vi "梦幻城堡C6~20界面.vi"() -> ()   [LabVIEW 2016, in "环境动力监测库.lvlib" / "UPS库.lvlib"]
uses:
  <vilib>/Utility/config.llb/NI_LVConfig.lvlib
panel:
  out "x+1":u32
  in  "解除告警":bool
  out "状态":T1
  out "通信":bool=TRUE
  out "串口":string
  in  "查看型号":bool
  out "关闭中":bool
  out "关机倒计时":i32
  out "UPS状态":T2
  in  "关机":bool
  in  "重开串口":bool
  # "V"
  # "输入电压"
  # "输出电压"
  # "V"
  # "输出电流"
  # "A"
  # "Hz"
  # "输入频率"
  # "电池电压"
  # "V"
  # "℃"
  # "UPS温度"
  # "%"
  # "电池容量百分比"
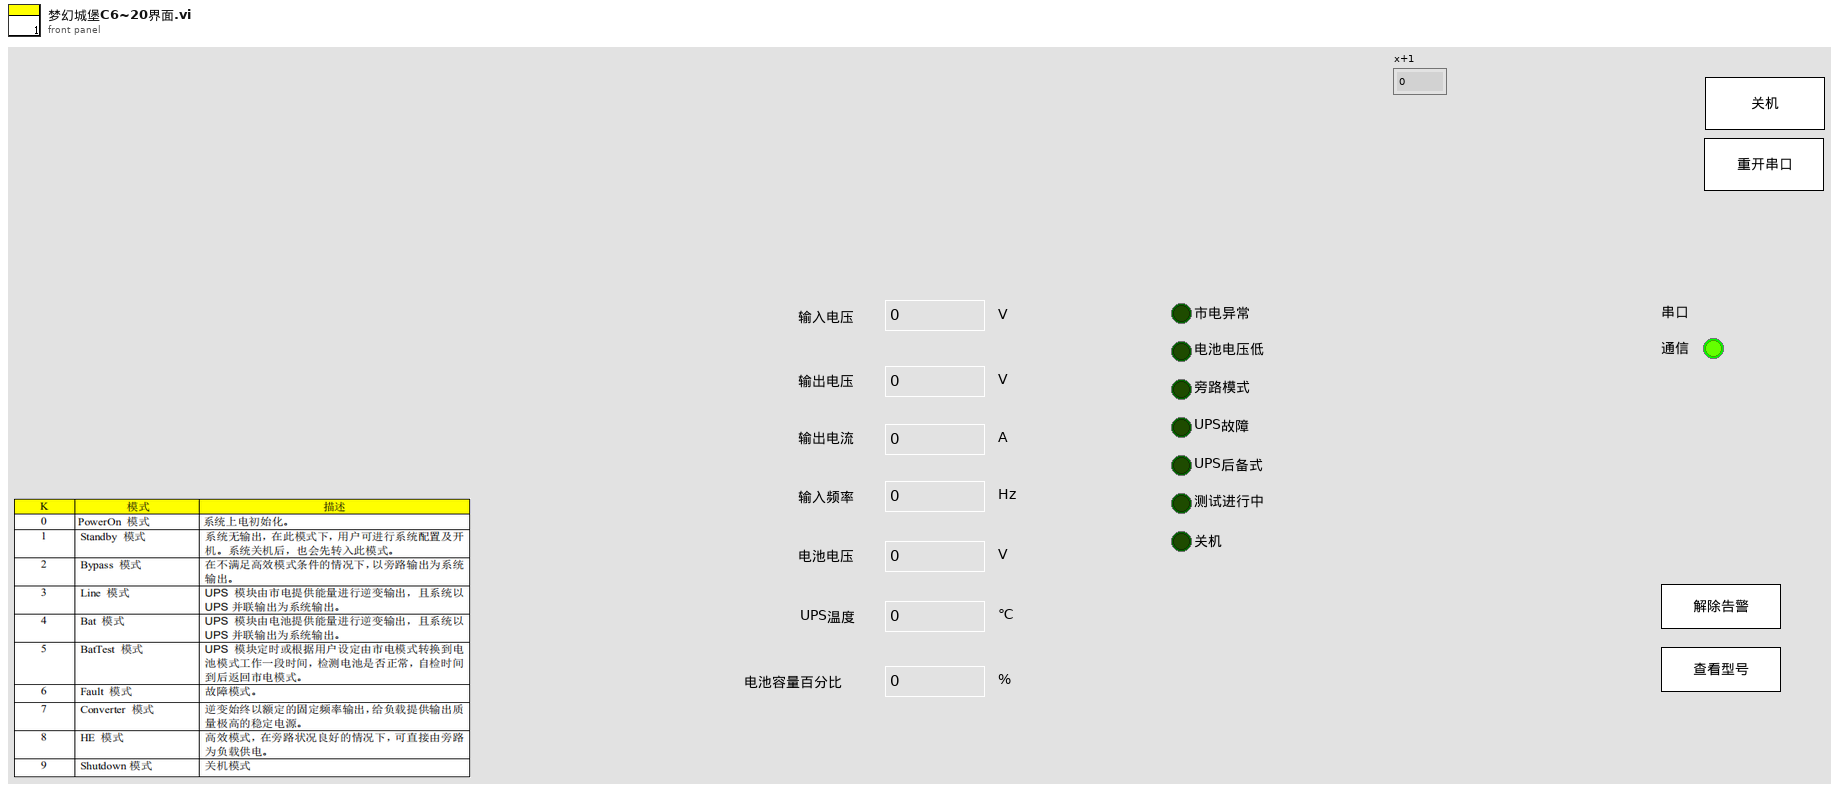
[diagram p1: front panel]
types:
  T1 = cluster{"I/P voltage":dbl, "O/P voltage":dbl, "O/P load %":dbl, "I/P frequency HZ":dbl, "Battery voltage":dbl, "Temperature":dbl, "CCC":dbl}
  T2 = cluster{"市电异常":bool, "电池电压低":bool, "旁路模式":bool, "UPS故障":bool, "UPS后备式":bool, "测试进行中":bool, "关机":bool, "保留":bool}
  T3 = cluster{"枚举":enum16{"open", "read", "write", "close"}, "写入缓冲区":string}
  T4 = cluster{"漏水监测输出":cluster{"漏水监测告警":bool, "告警内容":string}, "门禁监测输出":cluster{"门禁监测告警":bool, "告警内容":string}, "门禁监测输出2":cluster{"门禁监测告警":bool, "告警内容":string}, "温湿度监测输出":cluster{"温湿度监测告警":bool, "告警内容":string}, "烟雾监测输出":cluster{"烟雾监测告警":bool, "告警内容":string}, "空调监测输出":cluster{"空调监测告警":bool, "告警内容":string}, "自动重合闸输出":cluster{"自动重合闸告警":bool, "告警内容":string}, "红外入侵输出":cluster{"红外入侵告警":bool, "告警内容":string}, "振动输出":cluster{"振动告警":bool, "告警内容":string}, "UPS输出":cluster{"UPS告警":bool, "告警内容":string}, "蓄电池输出":cluster{"蓄电池告警":bool, "告警内容":string}, "蓄电池输出2":cluster{"蓄电池告警":bool, "告警内容":string}, "GPS输出":cluster{"定位告警":bool, "告警内容":string}, "北斗输出":cluster{"定位告警":bool, "告警内容":string}, "气象输出":cluster{"气象告警":bool, "告警内容":string}}
  T5 = cluster{"VISA resource name":refnum<visa-resource-name>, "Serial Config":cluster{"baud rate (9600)":u32, "stop bits (10: 1 bit)":u16, "parity (0:none)":enum16{"None", "Odd", "Even", "Mark", "Space"}, "data bits (8)":u16, "timeout (10sec)":u32}, "型号选择":enum16{"山特UPSC1~3", "山特UPSC6~20", "华为UPS2000-G-(1-3KVA)"}, "HW-UPS-2000 MB session":refnum<class "MB_Master.lvclass">, "连接方式":enum16{"串口", "TCP"}, "IP":string, "Port":string}
  T6 = typedef "NI_LVConfig.lvlib/Config Data RefNum.ctl" = refnum<k1>
  T7 = cluster{"输出功率R":dbl, "输出功率S":dbl, "输出功率T":dbl, "输出视在功率R":dbl, "输出视在功率S":dbl, "输出视在功率T":dbl, "总功率":dbl, "总视在功率":dbl, "输出电流R":dbl, "输出电流S":dbl, "输出电流T":dbl, "输出负载百分比":dbl, "U":string}
  T8 = cluster{"输入电压R":dbl, "输入电压S":dbl, "输入电压T":dbl, "输入频率":dbl, "输出电压R":dbl, "输出电压S":dbl, "输出电压T":dbl, "输出频率":dbl, "输出电流R":dbl, "输出电流S":dbl, "输出电流T":dbl, "Positive电池电压":dbl, "Negative电池电压":dbl, "温度":dbl, "电池剩余备用时间":dbl, "电池容量百分比":dbl, "系统模式":dbl, "电池测试状态":dbl, "故障代码":string, "告警":string}
  T9 = cluster{"市电":cluster{"状态":bool, "电压:":u16, "电流：":dbl, "详情  ":bool}, "UPS":cluster{"状态":bool, "输入电压:":sgl, "输出电压:":sgl, "电池电量:":u8, "电量":u16, "详情  ":bool}, "蓄电池12V":cluster{"状态":bool, "电压:":sgl, "电流:":sgl, "电池电量:":u8, "电量":u16, "详情  ":bool}, "蓄电池24V":cluster{"状态":bool, "电压:":sgl, "电流:":sgl, "电池电量:":u8, "电量":u16, "详情  ":bool}}
  T10 = cluster{"[0]":bool, "[1]":bool, "[2]":bool, "[3]":bool, "[4]":bool, "[5]":bool, "[6]":bool, "[7]":bool}
  T11 = enum32{"Bad", "Idle", "Run top level", "Running"}
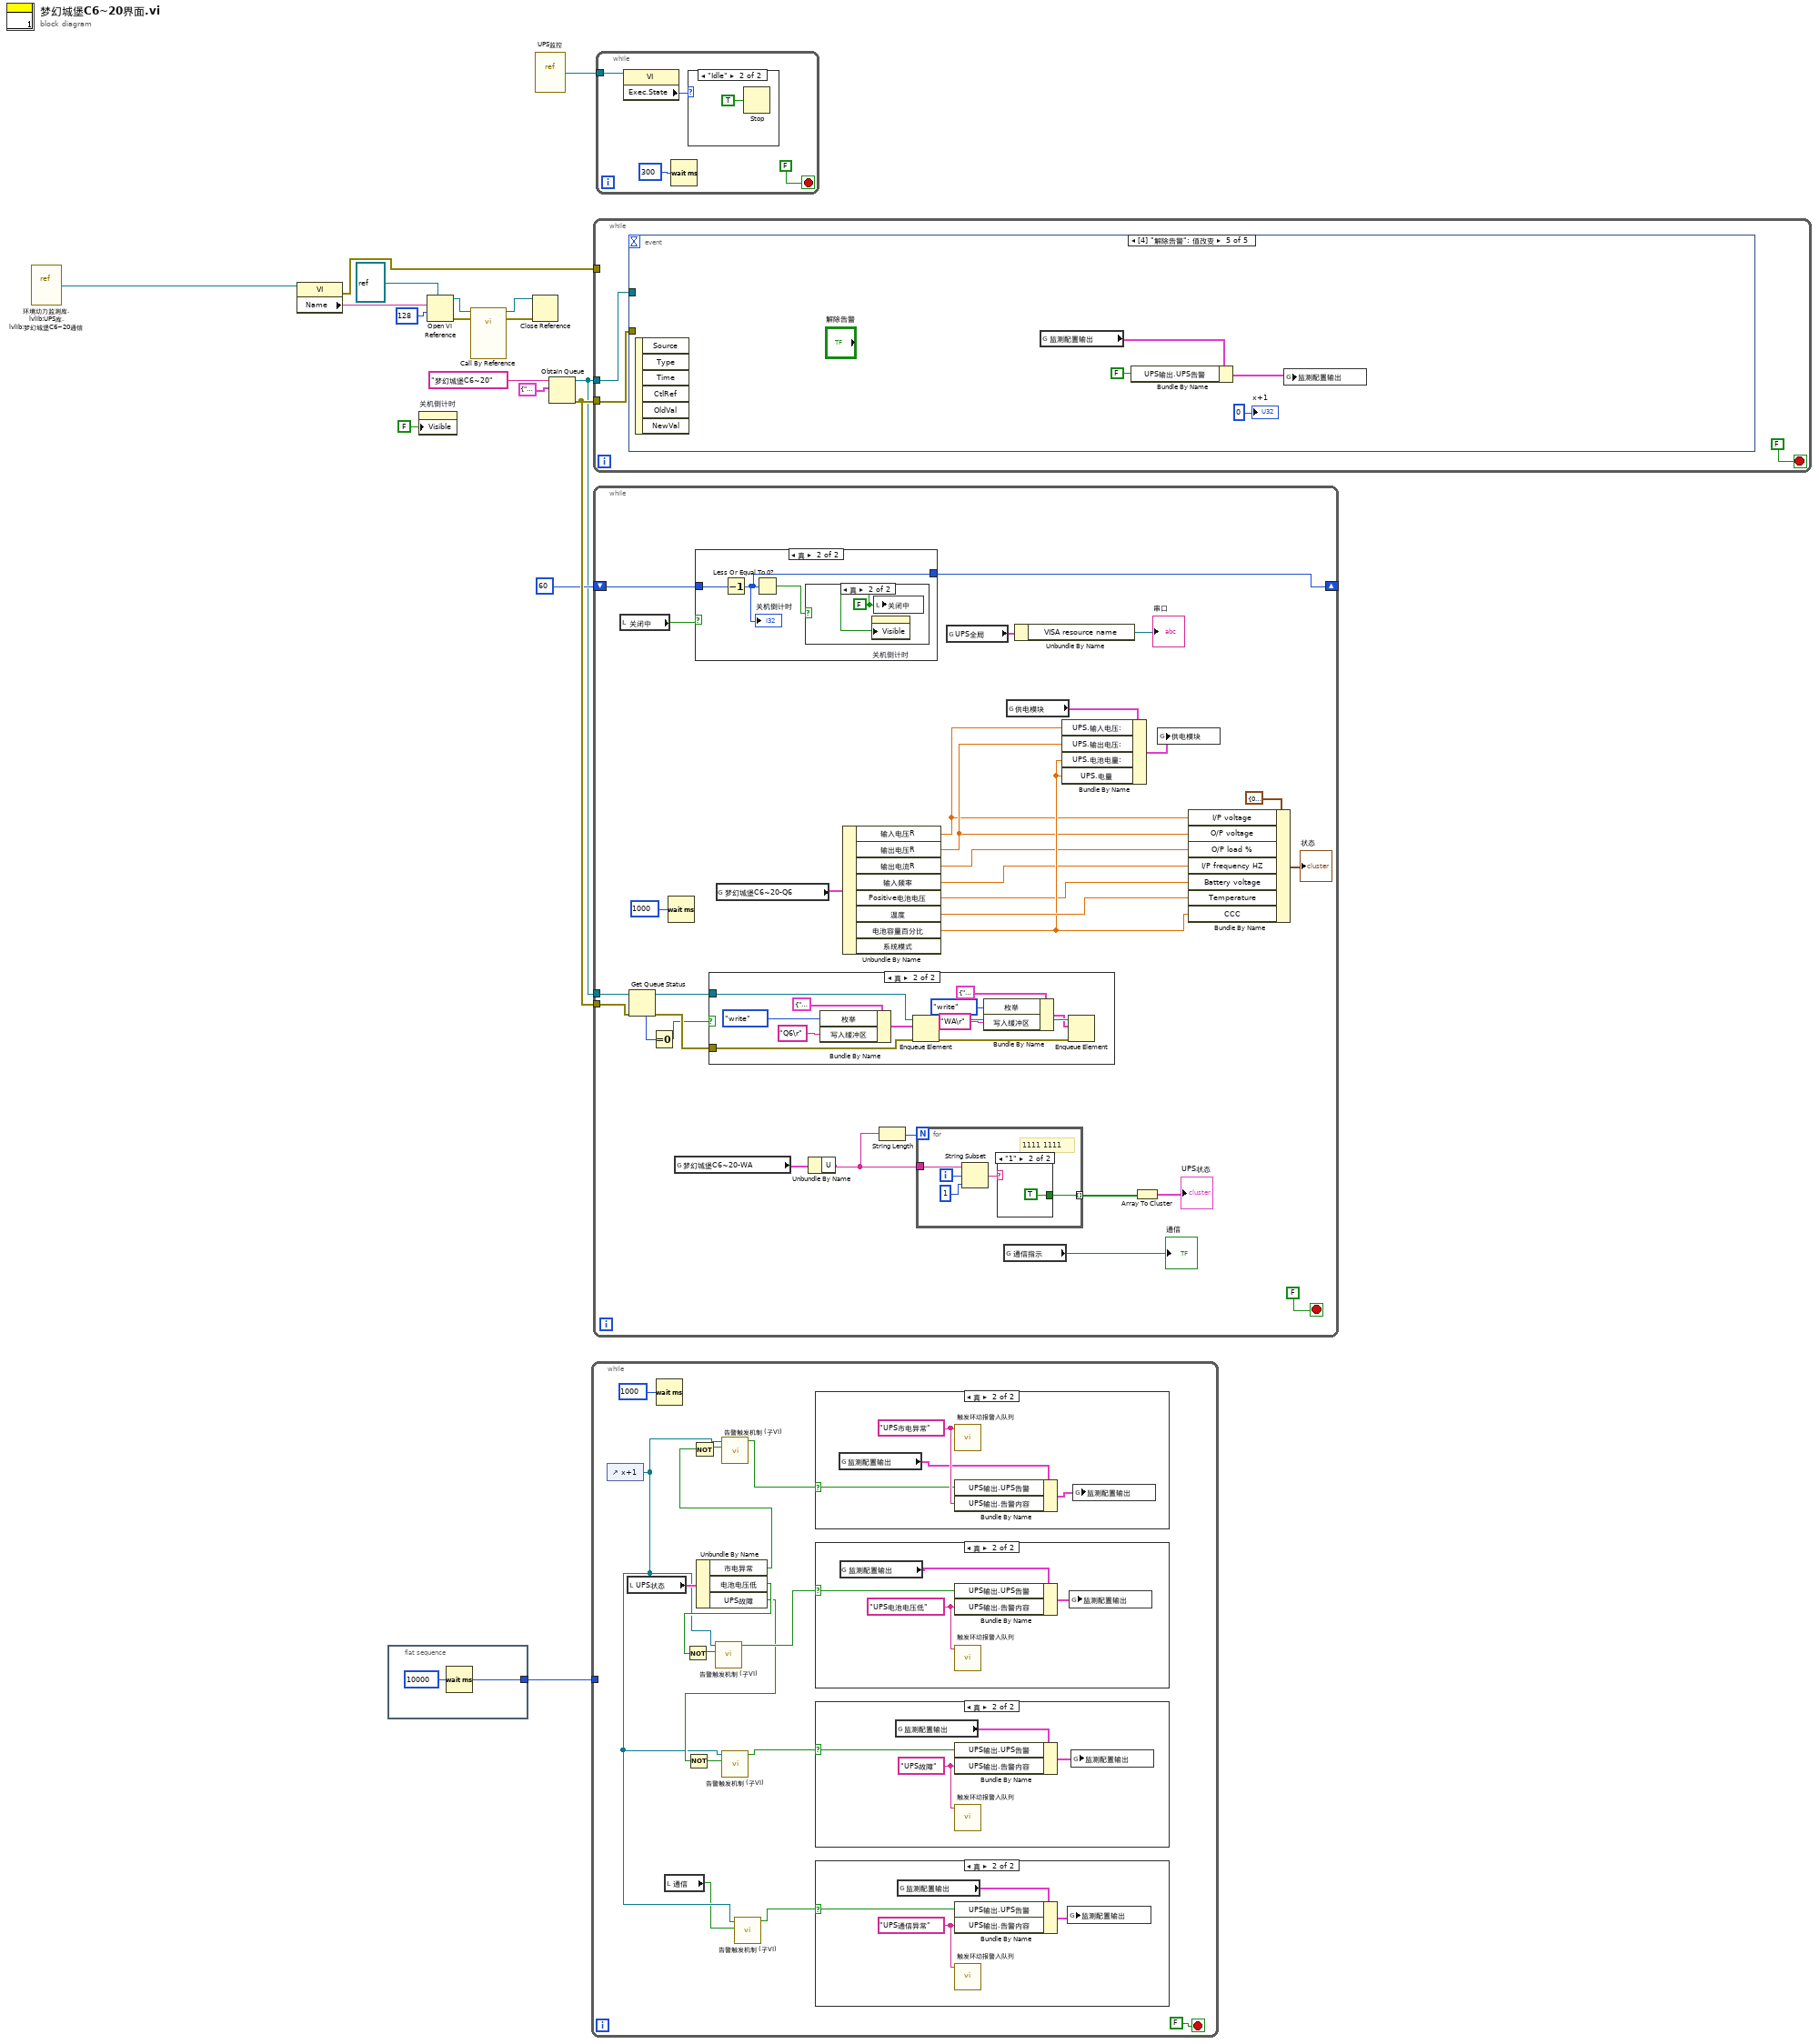
[diagram p0: block diagram]
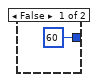
[diagram p7: hidden frame]
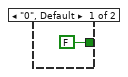
[diagram p9: hidden frame]
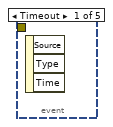
[diagram p11: hidden frame]
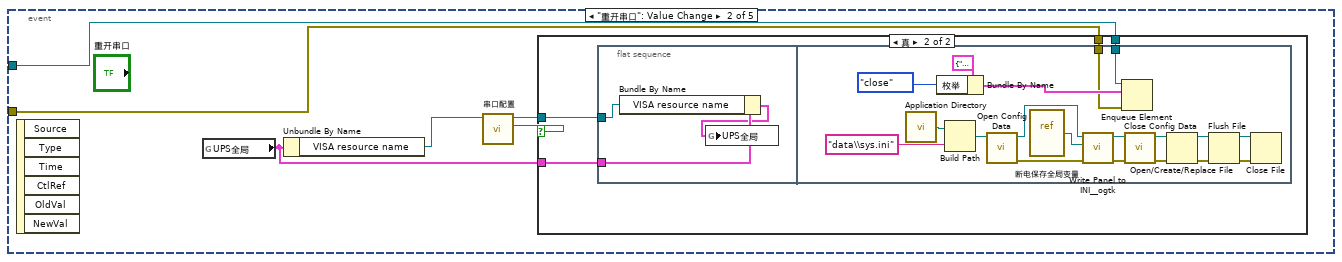
[diagram p12: hidden frame]
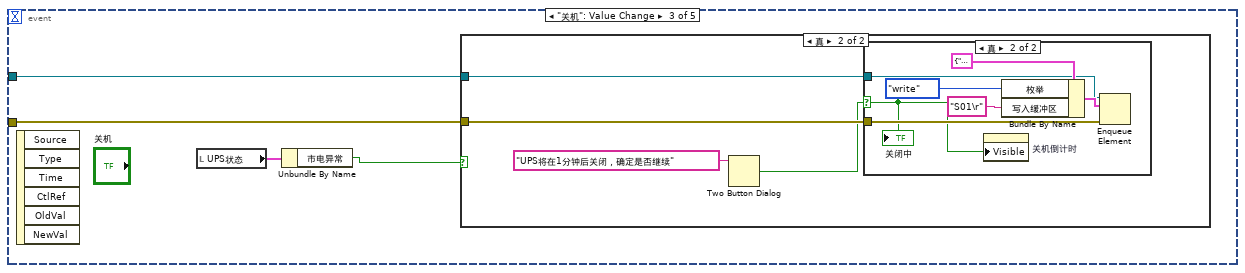
[diagram p14: hidden frame]
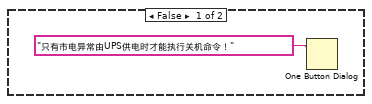
[diagram p15: hidden frame]
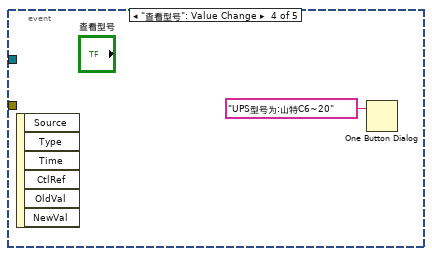
[diagram p17: hidden frame]
diagram:
  n1 = vi-ref "环境动力监测库.lvlib:UPS库.lvlib:梦幻城堡C6~20通信.vi"() -> (w10:refnum<vi>)
  n2 = property class="VI"(reference=w10) -> (error out=w4:errorcluster, "Name"=w11:string)  [unwired: 1 in, 1 out]
  n3 = flat-sequence {
    tunnel: [w18] -> w1
    frame #0 {
      n4 = Wait (ms)(milliseconds to wait=u32 10000 ("等待时间（毫秒）")) -> (millisecond timer value=w18:u32)
    }
  }
  n5 = property on="关机倒计时" class="DigNum (严格)"("Visible"=FALSE ("可见")) -> ()  [unwired: 2 in, 2 out]
  n6 = Open VI Reference(type specifier VI Refnum (for type only)=refnum<vi> refnum, vi path=w11, options=128 ("选项")) -> (vi reference=w13:refnum<vi>, error out=w15:errorcluster)  [unwired: 3 in]
  n7 = call-by-ref "?"(reference=w13, error in=w15) -> (reference out=w17:refnum<vi>, error out=w16:errorcluster)  [unwired: 12 in]
  n8 = Close Reference(reference=w17, error in (no error)=w16) -> ()  [unwired: 1 out]
  n9 = vi-ref "UPS监控.vi"() -> (w2:refnum<vi>)
  n10 = Obtain Queue(name (unnamed)="梦幻城堡C6~20" ("名称（未命名）"), element data type=T3 {"枚举"=enum."open", "写入缓冲区"=""}) -> (queue out=w5:refnum<queue>, error out=w7:errorcluster)  [unwired: 3 in, 1 out]
  n11 = while {
    tunnel: w1 -> [_]
    stop <- FALSE stop-if-true
    n12 = control-ref of="x+1"() -> (w22:refnum<vi>)
    n13 = local read "UPS状态"() -> (w33:T2)
    n14 = Wait (ms)(milliseconds to wait=u32 1000 ("等待时间（毫秒）")) -> ()  [unwired: 1 out]
    n15 = local read "通信"() -> (w21:bool)
    n16 = Unbundle By Name(w33) -> ("市电异常"=w30:bool, "电池电压低"=w27:bool, "UPS故障"=w24:bool)
    n17 = Not(x=w27) -> (.not. x?=w28:bool)
    n18 = Not(x=w24) -> (.not. x?=w25:bool)
    n19 = Not(x=w30) -> (.not. x?=w31:bool)
    n20 = call "告警触发机制 (子VI).vi"("状态输出"=w28, "Digital输入"=w22) -> ("触发告警"=w26:bool)  [unwired: 8 in, 1 out]
    n21 = call "告警触发机制 (子VI).vi"("状态输出"=w31, "Digital输入"=w22) -> ("触发告警"=w29:bool)  [unwired: 8 in, 1 out]
    n22 = call "告警触发机制 (子VI).vi"("状态输出"=w25, "Digital输入"=w22) -> ("触发告警"=w23:bool)  [unwired: 8 in, 1 out]
    n23 = call "告警触发机制 (子VI).vi"("状态输出"=w21, "Digital输入"=w22) -> ("触发告警"=w20:bool)  [unwired: 8 in, 1 out]
    n24 = case shown="真" w29 {
      selector: w29 -> [_ w49]
      frame False {
      }
      frame True {
        w50 = "UPS市电异常" ("报警内容")
        n25 = global read "内部交互全局变量.vi" "监测配置输出"() -> (w48:T4)
        n26 = call "触发环动报警入队列.vi"("报警内容"=w50) -> ()  [unwired: 11 in]
        n27 = Bundle By Name(cluster=w48, "UPS输出.UPS告警"=w49, "UPS输出.告警内容"=w50) -> (w47:T4)
        n28 = global write "内部交互全局变量.vi" "监测配置输出"(w47) -> ()
      }
    }
    n29 = case shown="真" w26 {
      selector: w26 -> [_ w45]
      frame False {
      }
      frame True {
        w46 = "UPS电池电压低" ("报警内容")
        n30 = global read "内部交互全局变量.vi" "监测配置输出"() -> (w44:T4)
        n31 = Bundle By Name(cluster=w44, "UPS输出.UPS告警"=w45, "UPS输出.告警内容"=w46) -> (w43:T4)
        n32 = call "触发环动报警入队列.vi"("报警内容"=w46) -> ()  [unwired: 11 in]
        n33 = global write "内部交互全局变量.vi" "监测配置输出"(w43) -> ()
      }
    }
    n34 = case shown="真" w23 {
      selector: w23 -> [_ w41]
      frame False {
      }
      frame True {
        w42 = "UPS故障" ("报警内容")
        n35 = global read "内部交互全局变量.vi" "监测配置输出"() -> (w40:T4)
        n36 = Bundle By Name(cluster=w40, "UPS输出.UPS告警"=w41, "UPS输出.告警内容"=w42) -> (w39:T4)
        n37 = call "触发环动报警入队列.vi"("报警内容"=w42) -> ()  [unwired: 11 in]
        n38 = global write "内部交互全局变量.vi" "监测配置输出"(w39) -> ()
      }
    }
    n39 = case shown="真" w20 {
      selector: w20 -> [_ w37]
      frame False {
      }
      frame True {
        w38 = "UPS通信异常" ("报警内容")
        n40 = global read "内部交互全局变量.vi" "监测配置输出"() -> (w35:T4)
        n41 = Bundle By Name(cluster=w35, "UPS输出.UPS告警"=w37, "UPS输出.告警内容"=w38) -> (w36:T4)
        n42 = call "触发环动报警入队列.vi"("报警内容"=w38) -> ()  [unwired: 11 in]
        n43 = global write "内部交互全局变量.vi" "监测配置输出"(w36) -> ()
      }
    }
  }
  n44 = while {
    tunnel: w7 -> [w52]
    tunnel: w5 -> [w51]
    tunnel: w4 -> [_]
    stop <- FALSE stop-if-true
    n45 = event shown="[4] \"解除告警\": 值改变" {
      selector: _ -> [_ _ _ _ _]
      dyn-events: _ -> [_ _ _ _ _]
      timeout: _ -> [_ _ _ _ _]
      tunnel: w52 -> [_ w56 w88 _ _]
      tunnel: w51 -> [_ w57 w89 _ _]
      event Timeout {
        n46 = event-data() -> ()  [unwired: 1 in, 3 out]
      }
      event "重开串口": Value Change {
        n47 = event-data() -> ()  [unwired: 1 in, 6 out]
        n48 = global read "断电保存全局变量.vi" "UPS全局"() -> (w54:T5)
        n49 = Unbundle By Name(w54) -> ("VISA resource name"=w55:refnum<visa-resource-name>)
        n50 = call "串口配置.vi"("请选择串口:"=w55) -> ("确认 2"=w59:bool, "请选择串口: 2"=w58:refnum<visa-resource-name>)  [unwired: 9 in]
        n51 = case shown="真" w59 {
          tunnel: w58 -> [_ w63]
          tunnel: w57 -> [_ w62]
          tunnel: w56 -> [_ w61]
          tunnel: w54 -> [_ w60]
          frame False {
          }
          frame True {
            n52 = flat-sequence {
              tunnel: w63 -> [w65]
              tunnel: w60 -> [w66]
              tunnel: w62 -> [w68]
              tunnel: w61 -> [w67]
              frame #0 {
                n53 = Bundle By Name(cluster=w66, "VISA resource name"=w65) -> (w64:T5)
                n54 = global write "断电保存全局变量.vi" "UPS全局"(w64) -> ()
              }
              frame #1 {
                n55 = call <vilib>:"Application Directory.vi"() -> ("Application Directory"=w73:path)
                n56 = Bundle By Name(cluster=T3 {"枚举"=enum."open", "写入缓冲区"=""}, "枚举"=enum16{"open", "read", "write", "close"}."close" ("元素")) -> (w71:T3)
                n57 = Build Path(base path=w73, name or relative path="data\\sys.ini" ("名称或相对路径")) -> (appended path=w74:path)
                n58 = call <vilib>:"Open Config Data.vi"("configuration file path"=w74) -> ("error out"=w78:errorcluster, "refnum"=w75:T6)  [unwired: 8 in, 1 out]
                n59 = vi-ref "断电保存全局变量.vi"() -> (w76:refnum<vi>)
                n60 = call <userlib>:"Write Panel to INI__ogtk.vi"("error in (no error)"=w78, "VI ref"=w76, "refnum"=w75) -> ("error out"=w79:errorcluster, "refnum out"=w77:T6)  [unwired: 7 in]
                n61 = Enqueue Element(queue=w68, element=w71, error in (no error)=w67) -> ()  [unwired: 1 in, 3 out]
                n62 = call <vilib>:"Close Config Data.vi"("error in (no error)"=w79, "refnum"=w77) -> ("error out"=w84:errorcluster, "file path"=w85:path)  [unwired: 8 in]
                n63 = Open/Create/Replace File(file path (use dialog)=w85, error in=w84) -> (refnum out=w81:refnum<file>, error out=w80:errorcluster)  [unwired: 4 in, 1 out]
                n64 = Flush File(refnum=w81, error in=w80) -> (refnum out=w82:refnum<file>, error out=w83:errorcluster)
                n65 = Close File(refnum=w82, error in=w83) -> ()  [unwired: 2 out]
              }
            }
          }
        }
      }
      event "关机": Value Change {
        n66 = event-data() -> ()  [unwired: 1 in, 6 out]
        n67 = local read "UPS状态"() -> (w87:T2)
        n68 = Unbundle By Name(w87) -> ("市电异常"=w86:bool)
        n69 = case shown="真" w86 {
          tunnel: w89 -> [_ w94]
          tunnel: w88 -> [_ w93]
          frame False {
            n70 = One Button Dialog(message="只有市电异常由UPS供电时才能执行关机命令！" ("消息")) -> ()  [unwired: 1 in, 1 out]
          }
          frame True {
            n71 = Two Button Dialog(message="UPS将在1分钟后关闭，确定是否继续" ("消息")) -> (T button?=w91:bool)  [unwired: 2 in]
            n72 = case shown="真" w91 {
              selector: w91 -> [_ w95]
              tunnel: w94 -> [_ w98]
              tunnel: w93 -> [_ w97]
              frame False {
              }
              frame True {
                n73 = property on="关机倒计时" class="DigNum (严格)"("Visible"=w95) -> ()  [unwired: 2 in, 2 out]
                n74 = Bundle By Name(cluster=T3 {"枚举"=enum."open", "写入缓冲区"=""}, "枚举"=enum16{"open", "read", "write", "close"}."write", "写入缓冲区"="S01\r") -> (w99:T3)
                n75 = Enqueue Element(queue=w98, element=w99, error in (no error)=w97) -> ()  [unwired: 1 in, 3 out]
                "关闭中" <- w95
              }
            }
          }
        }
      }
      event "查看型号": Value Change {
        n76 = event-data() -> ()  [unwired: 1 in, 6 out]
        n77 = One Button Dialog(message="UPS型号为:山特C6~20" ("消息")) -> ()  [unwired: 1 in, 1 out]
      }
      event "解除告警": Value Change {
        n78 = event-data() -> ()  [unwired: 1 in, 6 out]
        n79 = global read "内部交互全局变量.vi" "监测配置输出"() -> (w104:T4)
        n80 = Bundle By Name(cluster=w104, "UPS输出.UPS告警"=FALSE) -> (w103:T4)
        n81 = global write "内部交互全局变量.vi" "监测配置输出"(w103) -> ()
        "x+1" <- u32 0 ("x+1")
      }
    }
  }
  n82 = while {
    tunnel: w5 -> [w134]
    tunnel: w7 -> [w133]
    shift-right: [w123] -> _
    shift-left: 60 -> [w124]
    stop <- FALSE stop-if-true
    n83 = local read "关闭中"() -> (w125:bool)
    n84 = Get Queue Status(queue=w134, error in (no error)=w133) -> (queue out=w132:refnum<queue>, error out=w131:errorcluster, # elements in queue=w130:i32)  [unwired: 1 in, 5 out]
    n85 = Equal To 0?(x=w130) -> (x = 0?=w129:bool)
    n86 = Wait (ms)(milliseconds to wait=u32 1000 ("等待时间（毫秒）")) -> ()  [unwired: 1 out]
    n87 = global read "UPS内部交互全局.vi" "梦幻城堡C6~20-WA"() -> (w128:T7)
    n88 = case shown="真" w125 {
      tunnel: w124 -> [_ w141]
      tunnel: [60 w140] -> w123
      frame False {
      }
      frame True {
        n89 = Decrement(x=w141) -> (x-1=w140:i32)
        "关机倒计时" <- w140
        n90 = Less Or Equal To 0?(x=w140) -> (x <= 0?=w139:bool)
        n91 = case shown="真" w139 {
          frame False {
          }
          frame True {
            w142 = FALSE ("关闭中")
            n92 = property on="关机倒计时" class="DigNum (严格)"("Visible"=w142) -> ()  [unwired: 2 in, 2 out]
            n93 = local write "关闭中"(w142) -> ()
          }
        }
      }
    }
    n94 = case shown="真" w129 {
      tunnel: w132 -> [_ w157]
      tunnel: w131 -> [_ w156]
      frame False {
      }
      frame True {
        n95 = Bundle By Name(cluster=T3 {"枚举"=enum."open", "写入缓冲区"=""}, "枚举"=enum16{"open", "read", "write", "close"}."write", "写入缓冲区"="Q6\r") -> (w160:T3)
        n96 = Enqueue Element(queue=w157, element=w160, error in (no error)=w156) -> (queue out=w155:refnum<queue>, error out=w154:errorcluster)  [unwired: 1 in, 1 out]
        n97 = Bundle By Name(cluster=T3 {"枚举"=enum."open", "写入缓冲区"=""}, "枚举"=enum16{"open", "read", "write", "close"}."write", "写入缓冲区"="WA\r") -> (w150:T3)
        n98 = Enqueue Element(queue=w155, element=w150, error in (no error)=w154) -> ()  [unwired: 1 in, 3 out]
      }
    }
    n99 = global read "UPS内部交互全局.vi" "梦幻城堡C6~20-Q6"() -> (w135:T8)
    n100 = Unbundle By Name(w128) -> ("U"=w126:string)
    n101 = Unbundle By Name(w135) -> ("输入电压R"=w109:dbl, "输出电压R"=w110:dbl, "输出电流R"=w111:dbl, "输入频率"=w112:dbl, "Positive电池电压"=w113:dbl, "温度"=w115:dbl, "电池容量百分比"=w114:dbl)  [unwired: 1 out]
    n102 = String Length(string=w126) -> (length=w127:i32)
    n103 = for {
      N: w127 -> [_]
      tunnel: w126 -> [w147]
      tunnel: [w143] -> w119 mode=indexing
      i -> [w145]
      # "1111 1111"
      n104 = String Subset(string=w147, offset (0)=w145, length (rest)=1 ("长度（剩余）")) -> (substring=w144:string)
      n105 = case shown="\"1\"" w144 {
        tunnel: [FALSE TRUE] -> w143
        frame "0", Default {
        }
        frame "1" {
        }
      }
    }
    n106 = global read "断电保存全局变量.vi" "UPS全局"() -> (w108:T5)
    n107 = global read "UPS内部交互全局.vi" "通信指示"() -> (→"通信":bool)
    n108 = global read "内部交互全局变量.vi" "供电模块"() -> (w121:T9)
    n109 = Unbundle By Name(w108) -> ("VISA resource name"=→"串口":refnum<visa-resource-name>)
    n110 = Bundle By Name(cluster=w121, "UPS.输入电压:"=w109, "UPS.输出电压:"=w110, "UPS.电池电量:"=w114, "UPS.电量"=w114) -> (w120:T9)
    n111 = Array To Cluster(array=w119) -> (cluster=→"UPS状态":T10)
    n112 = global write "内部交互全局变量.vi" "供电模块"(w120) -> ()
    n113 = Bundle By Name(cluster=T1 {"I/P voltage"=0.0, "O/P voltage"=0.0, "O/P load %"=0.0, "I/P frequency HZ"=0.0, "Battery voltage"=0.0, "Temperature"=0.0, "CCC"=0.0} ("状态"), "I/P voltage"=w109, "O/P voltage"=w110, "O/P load %"=w111, "I/P frequency HZ"=w112, "Battery voltage"=w113, "Temperature"=w115, "CCC"=w114) -> (→"状态":T1)
  }
  n114 = while {
    tunnel: w2 -> [w165]
    stop <- FALSE stop-if-true
    n115 = property class="VI"(reference=w165) -> ("Exec.State"=w164:T11)  [unwired: 1 in, 2 out]
    n116 = Wait (ms)(milliseconds to wait=u32 300 ("等待时间（毫秒）")) -> ()  [unwired: 1 out]
    n117 = case shown="\"Idle\"" w164 {
      frame "Bad", Default {
      }
      frame "Idle" {
        n118 = Stop(stop? (T)=TRUE ("停止？(T)")) -> ()
      }
    }
  }
